vi "Vision Processing.vi"(4 "error in (no error)":errorcluster, 6 "CameraDevRef":T1) -> ()   [LabVIEW 2011]
uses:
  <vilib>/Rock Robotics/WPI/Camera/WPI_CameraDevRef.ctl
  Robot Global Data.vi
  <vilib>/vision/NI_Vision_Development_Module.lvlib
panel:
  in  "Scale":dbl=0.85
  in  "Minimum Power":dbl=0.23
  out "Aspect Ratio":dbl[](array[numeric])
  out "Offset":dbl
  in  "Max Distance for 1 hoop":dbl=8.0
  out "Raw Turret":dbl
  in  "Run Calculations":bool=TRUE
  out "Target X Coord":dbl
  out "Target Distance":dbl
  out "Target Y Coord":dbl
  out "Distance Array":dbl[](array[numeric])
  in  "Dead Band":dbl=0.09
  out "Number of Rectangles Visible":dbl
  out "Y Position Array":dbl[](array[numeric])
  out "X Position Array":dbl[](array[numeric])
  in  "View":bool
  out "Target Info":T2(array[cluster])
  in  "Area Size Limit":i32=444
  in  "Particle Count Limit":i32=8
  in  "Score Limits":T3={"Rect Coverage"=76.0, "Aspect Ratio"=40.0, "X Edge Strength"=40.0, "Y Edge Strength"=60.0}
  in  "Processing":enum32{"Color", "Intensity", "Intensity Open"}(tab)=enum."Intensity"
  in  "Luminance":i32=255
  in  "Saturation":i32=255
  in  "Hue":i32(knob)=65 scale=0.0..255.0
  in  "Margins":cluster{"Hue":i32, "Sat":i32, "Lum":i32}={"Hue"=20, "Sat"=27, "Lum"=30} {"Sat" scale=0.0..40.0; "Lum" scale=0.0..40.0; "Hue" scale=0.0..40.0}
  in  "Range":cluster{"Lower value":sgl, "Upper value":sgl}={"Lower value"=107.17391, "Upper value"=255.0} {"Lower value" scale=0.0..255.0; "Upper value" scale=0.0..255.0}
  in  "Range":cluster{"Lower value":sgl, "Upper value":sgl}={"Lower value"=123.804344, "Upper value"=255.0} {"Lower value" scale=0.0..255.0; "Upper value" scale=0.0..255.0}
  in  "View":bool
  out "Processed Image":T4(plugin-control)
  out "Original Image":T4(plugin-control)
  # "Instructions:\nProcessing the reflective tape that is illuminated by a ring light can be based\non color or light intensity.\nParticles within the image are scored by rectangle coverage, aspect ratio, and\nfor being hollow with a bold edge. A particle is considered a target if all scores\nare above the score limits. Particles can be annotated -- surrounded by\na rectangle and scores drawn to the left .\nTo control the number of particles being scored, use the count limit and the size\nlimit."
  # "(in)"
  # "To debug, Enable using the View button.\nFor color processing, you can click in the image to select the color for processing."
  # "Enable by clicking the View button.\nGreen scores are above the limit, orange are below. Inner/outer rect\nindicates all passed."
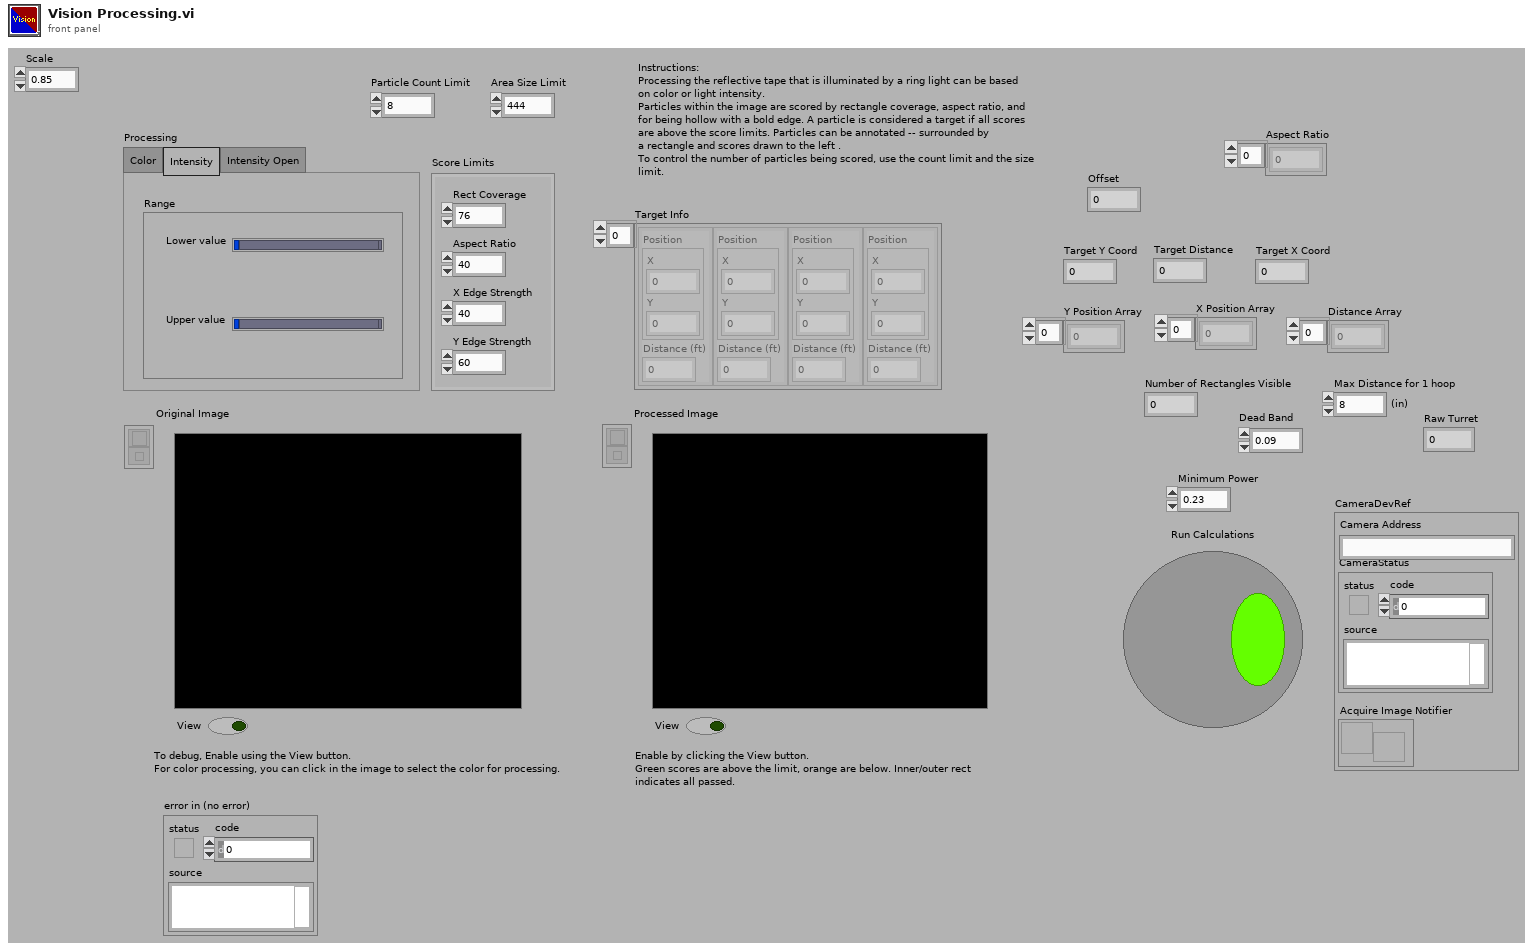
[diagram p1: front panel]
types:
  T1 = typedef "WPI_CameraDevRef.ctl" = cluster{"Camera Address":string, "CameraStatus":errorcluster, "Acquire Image Notifier":refnum<notifier>}
  T2 = cluster{"Position":cluster{"X":dbl, "Y":dbl}, "Distance (ft)":dbl}[]
  T3 = cluster{"Rect Coverage":dbl, "Aspect Ratio":dbl, "X Edge Strength":dbl, "Y Edge Strength":dbl}
  T4 = typedef "IMAQ Image.ctl" = refnum<image>
  T5 = typedef "Image Type" = u32
  T6 = enum32{"AutoM", "Close", "Dilate", "Erode", "Gradient", "Gradient out", "Gradient in", "Hit miss", "Open", "PClose", "POpen", "Thick", "Thin"}
  T7 = typedef "WPI_CameraImageSize.ctl" = enum16{"640x480", "320x240", "160x120"}
  T8 = cluster{"fps":i32, "compression":i32, "Image Size":T7}
  T9 = cluster{cluster{"Left":dbl, "Top":dbl, "Right":dbl, "Bottom":dbl}, dbl[]}[]
  T10 = cluster{"Left":dbl, "Top":dbl, "Right":dbl, "Bottom":dbl}
  T11 = cluster{"Target Center (-1 to 1)":cluster{"X":dbl, "Y":dbl}, "Distance (ft)":dbl}
  T12 = cluster{"Target Center (-1 to 1)":cluster{"X":dbl, "Y":dbl}, "Distance (ft)":dbl}[]
  T13 = typedef "WPI_JoystickDevRef.ctl" = cluster{"Device":T14}
  T14 = typedef "WPI_JoystickDeviceEnum.ctl" = enum16{"USB 1", "USB 2", "USB 3", "USB 4", "Kinect 1", "Kinect 2"}
  T15 = typedef "WPI_JoystickButtonState.ctl" = cluster{"Button 1":bool, "Button 2":bool, "Button 3":bool, "Button 4":bool, "Button 5":bool, "Button 6":bool, "Button 7":bool, "Button 8":bool, "Button 9":bool, "Button 10":bool, "Button 11":bool, "Button 12":bool}
  T16 = cluster{"axis 1 (x)":dbl, "axis 2 (y)":dbl, "axis 3 (throttle)":dbl, "axis 4":dbl, "axis 5":dbl, "axis 6":dbl}
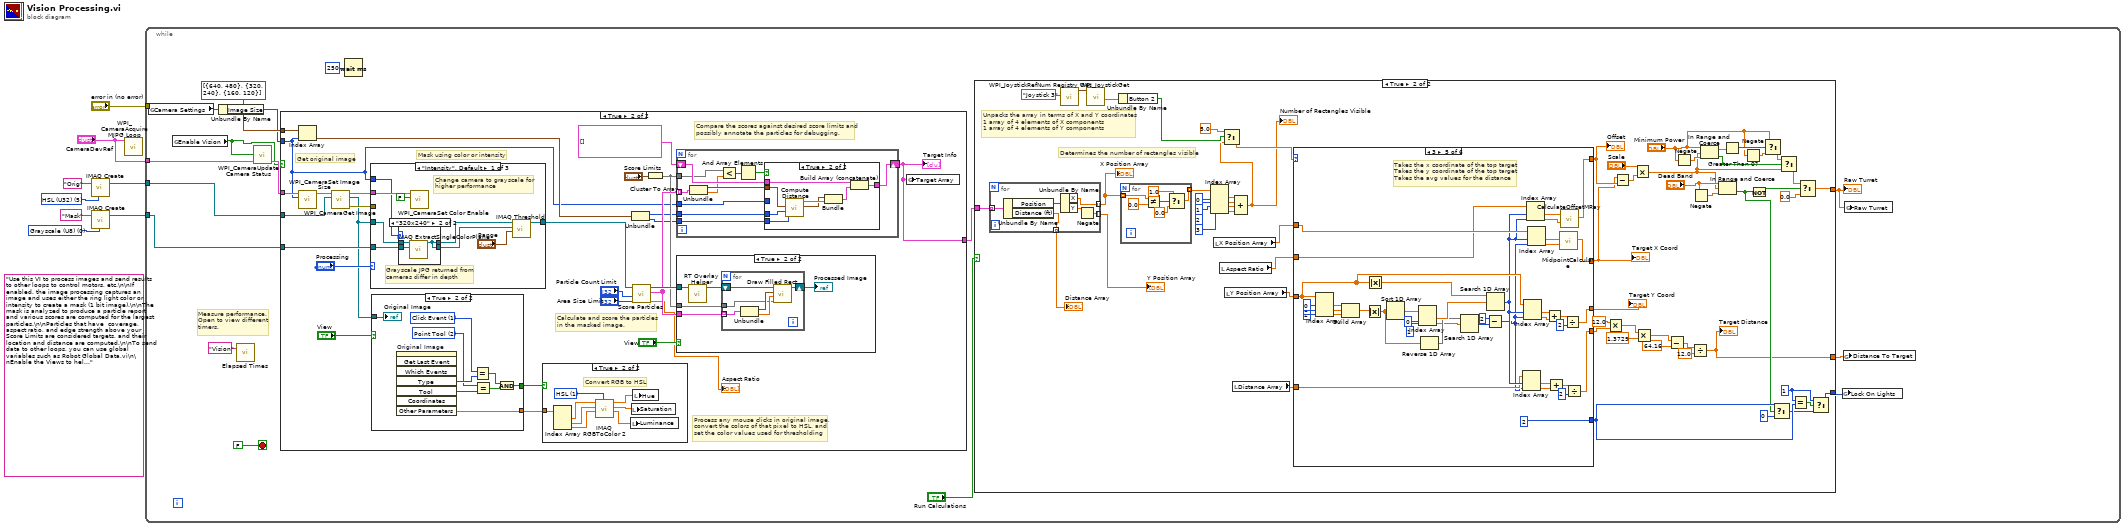
[diagram p0: block diagram]
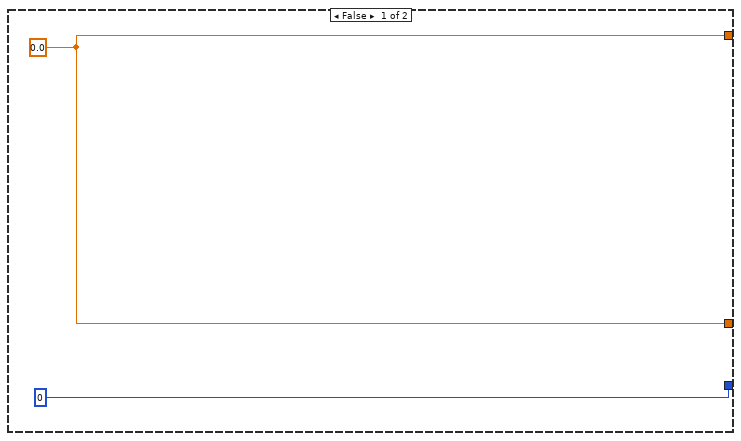
[diagram p2: hidden frame]
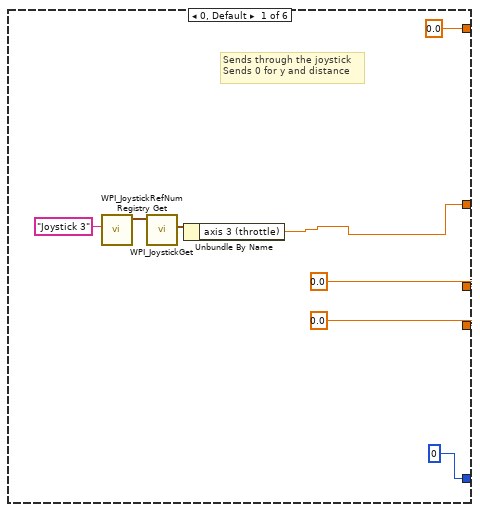
[diagram p3: hidden frame]
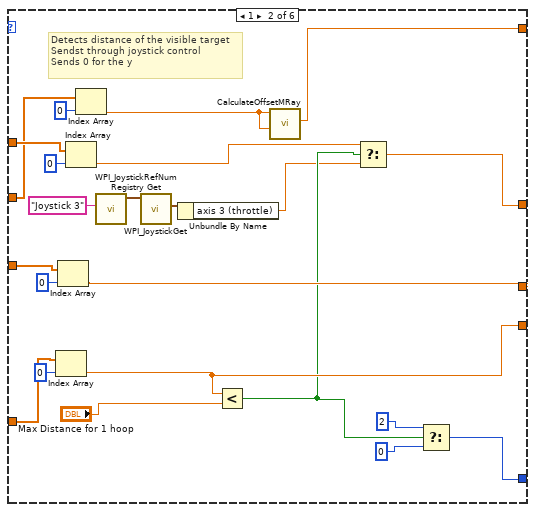
[diagram p4: hidden frame]
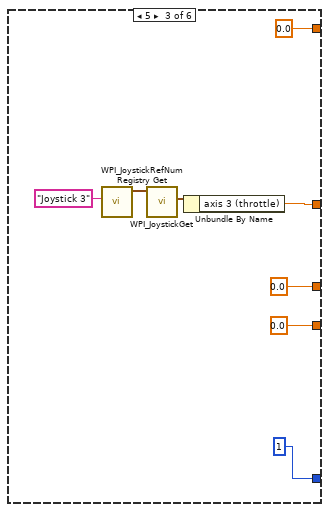
[diagram p5: hidden frame]
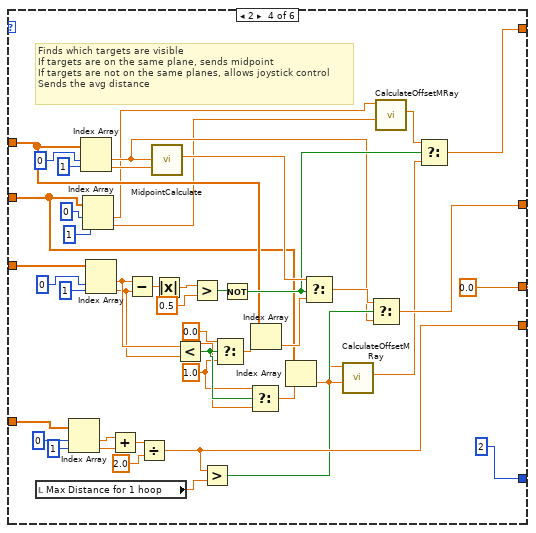
[diagram p6: hidden frame]
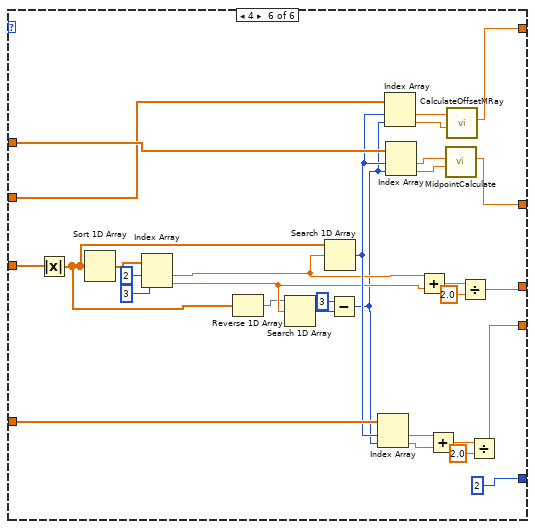
[diagram p7: hidden frame]
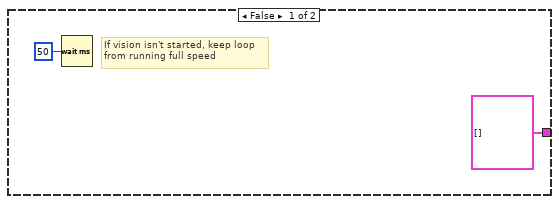
[diagram p8: hidden frame]
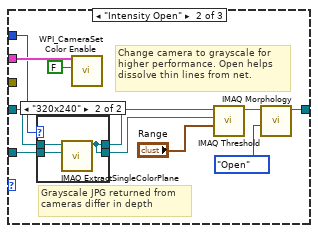
[diagram p11: hidden frame]
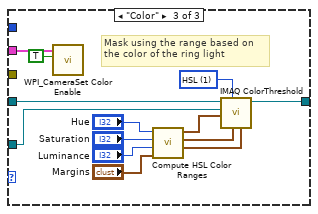
[diagram p13: hidden frame]
diagram:
  w3 = T5 0 items=["Grayscale (U8)", "Grayscale (I16)", "Grayscale (SGL)", "Complex (CSG)", "RGB (U32)", "HSL (U32)", "RGB (U64)", "Grayscale (U16)"] ("Image Type")
  (unwired) "Use this VI to process images and send results to other loops to control motors, etc.\n\nIf enabled, the image processing captures an image and uses either the ring light color or intensity to create a mask (1 bit image).\n\nThe mask is analyzed to produce a particle report and various scores are computed for the largest particles.\n\nParticles that have  coverage, aspect ratio, and edge strength above your Score Limits are considered targets, and their location and distance are computed.\n\nTo send data to other loops, you can use global variables such as Robot Global Data.vi\n\nEnable the Views to help debug color settings. Disable the View to speed up processing."
  w7 = T5 5 items=["Grayscale (U8)", "Grayscale (I16)", "Grayscale (SGL)", "Complex (CSG)", "RGB (U32)", "HSL (U32)", "RGB (U64)", "Grayscale (U16)"] ("Image Type")
  n1 = call "IMAQ Create"("Image Name"="Orig", "Image Type"=w7) -> ("New Image"=w6:T4)  [unwired: 2 in, 2 out]
  n2 = call "IMAQ Create"("Image Name"="Mask", "Image Type"=w3) -> ("New Image"=w1:T4)  [unwired: 2 in, 2 out]
  n3 = call <vilib>:"WPI_CameraAcquire MJPG Loop.vi"("CameraDevRef"="CameraDevRef") -> ()  [unwired: 11 in]
  n4 = while {
    tunnel: w6 -> [w23]
    tunnel: "CameraDevRef" -> [w22]
    tunnel: "error in (no error)" -> [_]
    tunnel: w1 -> [w18]
    stop <- FALSE stop-if-true
    # "Measure performance.\nOpen to view different\ntimers."
    n5 = global read "Robot Global Data.vi" "Camera Settings"() -> (w16:T8)
    n6 = global read "Robot Global Data.vi" "Enable Vision"() -> (w20:bool)
    n7 = Unbundle By Name(w16) -> ("Image Size"=w15:T7)
    n8 = call "Elapsed Times.vi"("Call Name"="Vision") -> ()  [unwired: 2 in, 1 out]
    n9 = call <vilib>:"WPI_CameraUpdate Camera Status.vi"("CameraDevRef In"=w22, "Enable Vision"=w20) -> ("CameraDevRef Out"=w21:T1)  [unwired: 3 in]
    n10 = case shown="True" w20 {
      tunnel: w23 -> [_ w271]
      tunnel: w21 -> [_ w267]
      tunnel: w18 -> [_ w258]
      tunnel: cluster{i32, i32}[] [{640, 480}, {320, 240}, {160, 120}] -> [_ w262]
      tunnel: w15 -> [_ w255]
      tunnel: [T2 [] w256] -> w14
      frame False {
        # "If vision isn't started, keep loop\nfrom running full speed"
        n11 = Wait (ms)(milliseconds to wait=u32 50) -> ()  [unwired: 1 out]
      }
      frame True {
        # "Compare the scores against desired score limits and\npossibly annotate the particles for debugging."
        # "Process any mouse clicks in original image,\nconvert the colors of that pixel to HSL, and\nset the color values used for thresholding"
        # "Calculate and score the particles\nin the masked image."
        # "Mask using color or intensity"
        # "Get original image"
        n12 = call <vilib>:"WPI_CameraSet Image Size.vi"("Image Size"=w255, "CameraDevRef"=w267) -> ("CameraDevRef Out"=w268:T1)  [unwired: 8 in, 1 out]
        n13 = Index Array(array=w262, index=w255) -> (element=w259:cluster{i32, i32})
        n14 = call <vilib>:"WPI_CameraGet Image.vi"("Image"=w271, "CameraDevRef"=w268) -> ("error out"=w269:errorcluster, "Image Out"=w257:T4, "CameraDevRef Out"=w270:T1)  [unwired: 7 in]
        n15 = case shown="\"Intensity\", Default" "Processing" {
          tunnel: w257 -> [w293 w305 w331]
          tunnel: [w296 w310 w330] -> w265
          tunnel: w270 -> [w294 w308 w321]
          tunnel: w269 -> [_ _ _]
          tunnel: w258 -> [w292 w306 w319]
          tunnel: w255 -> [w291 w307 _]
          frame "Intensity", Default {
            # "Grayscale JPG returned from\ncameras differ in depth"
            # "Change camera to grayscale for\nhigher performance"
            n16 = case shown="\"320x240\"" w291 {
              tunnel: w293 -> [w299 w302]
              tunnel: w292 -> [w298 w301]
              tunnel: [w299 w300] -> w290
              tunnel: [w298 w300] -> w289
              frame "640x480", Default {
              }
              frame "320x240" {
                n17 = call "IMAQ ExtractSingleColorPlane"("Image Dst"=w301, "Image Src"=w302) -> ("Image Dst Out"=w300:T4)  [unwired: 8 in, 1 out]
              }
            }
            n18 = call <vilib>:"WPI_CameraSet Color Enable.vi"("Color Enabled"=FALSE, "CameraDevRef"=w294) -> ()  [unwired: 8 in, 2 out]
            n19 = call "IMAQ Threshold"("Range"="Range", "Image Dst"=w289, "Image Src"=w290) -> ("Image Dst Out"=w296:T4)  [unwired: 3 in, 5 out]
          }
          frame "Intensity Open" {
            # "Grayscale JPG returned from\ncameras differ in depth"
            # "Change camera to grayscale for\nhigher performance. Open helps\ndissolve thin lines from net."
            n20 = case shown="\"320x240\"" w307 {
              tunnel: w305 -> [w315 w318]
              tunnel: w306 -> [w314 w317]
              tunnel: [w315 w316] -> w304
              tunnel: [w314 w316] -> w303
              frame "640x480", Default {
              }
              frame "320x240" {
                n21 = call "IMAQ ExtractSingleColorPlane"("Image Dst"=w317, "Image Src"=w318) -> ("Image Dst Out"=w316:T4)  [unwired: 8 in, 1 out]
              }
            }
            n22 = call <vilib>:"WPI_CameraSet Color Enable.vi"("Color Enabled"=FALSE, "CameraDevRef"=w308) -> ()  [unwired: 8 in, 2 out]
            n23 = call "IMAQ Threshold"("Range"="Range", "Image Dst"=w303, "Image Src"=w304) -> ("Image Dst Out"=w311:T4)  [unwired: 3 in, 5 out]
            n24 = call "IMAQ Morphology"("Operation"=T6."Open", "Image Src"=w311) -> ("Image Dst Out"=w310:T4)  [unwired: 8 in, 1 out]
          }
          frame "Color" {
            w329 = u16 1 items=["RGB", "HSL", "HSV", "HSI"] ("Color Mode")
            # "Mask using the range based on\nthe color of the ring light"
            n25 = call <vilib>:"WPI_CameraSet Color Enable.vi"("Color Enabled"=TRUE, "CameraDevRef"=w321) -> ()  [unwired: 8 in, 2 out]
            n26 = call "Compute HSL Color Ranges.vi"("Margins"="Margins", "Luminance"="Luminance", "Saturation"="Saturation", "Hue"="Hue") -> ("Lum Range"=w326:cluster{i32, i32}, "Sat Range"=w327:cluster{i32, i32}, "Hue Range"=w328:cluster{i32, i32})  [unwired: 5 in]
            n27 = call "IMAQ ColorThreshold"("Blue or Luma or Val or Inten Range"=w326, "Green or Sat Range"=w327, "Color Mode"=w329, "Red or Hue Range"=w328, "Image Dst"=w319, "Image Src"=w331) -> ("Image Dst Out"=w330:T4)  [unwired: 4 in, 1 out]
          }
        }
        n28 = case shown="True" "View" {
          tunnel: w257 -> [_ w351]
          tunnel: [_ w346] -> w264
          tunnel: [_ w343] -> w263
          frame False {
          }
          frame True {
            w344 = 2 items=["None", "Selection Tool", "Point Tool", "Line Tool", "Rectangle Tool", "Oval Tool", "Polygon Tool", "ClosedFreehandTool", "Annulus Tool", "Rotated Rectangle Tool", "Zoom Tool", "Pan Tool", "Polyline Tool", "Freehand Tool"] ("Tool")
            w345 = 1 items=["No Event"=0, "Click Event"=1, "Draw Event"=2, "Size Event"=4, "Scroll Event"=5, "Double Click Event"=8] ("Type")
            n29 = invoke on="Original Image" class="ImageControl" method="Get Last Event"() -> ("Type"=w347:i32, "Tool"=w350:i32, "Other Parameters"=w343:sgl[])  [unwired: 8 in, 5 out]
            n30 = Equal?(x=w345, y=w347) -> (x = y?=w348:bool)
            n31 = Equal?(x=w344, y=w350) -> (x = y?=w349:bool)
            n32 = And(x=w348, y=w349) -> (x .and. y?=w346:bool)
            "Original Image" <- w351
          }
        }
        n33 = case shown="True" w264 {
          tunnel: w263 -> [_ w288]
          frame False {
          }
          frame True {
            w287 = u16 1 items=["RGB", "HSL", "HSV", "HSI", "CIE L*a*b*", "CIE XYZ"] ("Color Mode")
            # "Convert RGB to HSL"
            n34 = Index Array(array=w288) -> (element #1=w286:sgl, element #2=w284:sgl, element #3=w282:sgl)  [unwired: 3 in]
            n35 = call "IMAQ RGBToColor 2"("Color Mode"=w287, "Blue value"=w282, "Green value"=w284, "Red value"=w286) -> ("Blue or Luma or Val or Inten or Z or b*value"=w281:dbl, "Green or Sat or Y or a* value"=w283:dbl, "Red or Hue or X or L* value"=w285:dbl)  [unwired: 4 in, 1 out]
            n36 = local write "Luminance"(w281) -> ()
            n37 = local write "Saturation"(w283) -> ()
            n38 = local write "Hue"(w285) -> ()
          }
        }
        n39 = Unbundle(w259) -> (w261:i32, w260:i32)
        n40 = call "Score Particles.vi"("Area Size Limit"="Area Size Limit", "Particle Count Limit"="Particle Count Limit", "Image Refnum in"=w265) -> ("Aspect Ratio"=→"Aspect Ratio":dbl[], "Scored Particle Info"=w276:T9, "Image Refnum out"=w279:T4)  [unwired: 6 in]
        n41 = Cluster To Array(cluster="Score Limits") -> (array=w274:dbl[])
        n42 = for {
          shift-right: [w361] -> w256
          shift-left: T2 [] -> [w362]
          tunnel: w261 -> [w360]
          tunnel: w276 -> [w358] mode=indexing
          tunnel: w274 -> [w353]
          tunnel: w255 -> [w357]
          tunnel: w260 -> [w352]
          n43 = Unbundle(w358) -> (w359:T10, w354:dbl[])
          n44 = Less?(x=w353, y=w354) -> (x < y?=w356:bool[])
          n45 = And Array Elements(Boolean array=w356) -> (logical AND=w355:bool)
          n46 = case shown="True" w355 {
            tunnel: w362 -> [w363 w371]
            tunnel: [w363 w370] -> w361
            tunnel: w359 -> [_ w366]
            tunnel: w360 -> [_ w368]
            tunnel: w357 -> [_ _]
            tunnel: w352 -> [_ w365]
            frame False {
            }
            frame True {
              n47 = call "Compute Distance.vi"("Y Image Resolution"=w365, "X Image Resolution"=w368, "Bounding Box"=w366) -> ("Target Center (-1 to 1)"=w364:cluster{"X":dbl, "Y":dbl}, "Distance (ft)"=w367:dbl)  [unwired: 7 in]
              n48 = Bundle("Target Center (-1 to 1)"=w364, "Distance (ft)"=w367) -> (w369:T11)  [unwired: 1 in]
              n49 = Build Array (concatenate)(w371, w369) -> (w370:T12)
            }
          }
        }
        "Target Info" <- w256
        n50 = case shown="True" "View" {
          tunnel: w279 -> [_ w333]
          tunnel: w276 -> [_ w335]
          tunnel: w274 -> [_ w334]
          frame False {
          }
          frame True {
            n51 = call "RT Overlay Helper.vi"("Refnum in"=w333) -> ("Refnum out"=w336:T4)  [unwired: 10 in]
            n52 = for {
              shift-right: [w341] -> w332
              shift-left: w336 -> [w342]
              tunnel: w335 -> [w338] mode=indexing
              tunnel: w334 -> [w337]
              n53 = Unbundle(w338) -> (w339:T10, w340:dbl[])
              n54 = call "Draw Filled Rect.vi"("Limits"=w337, "Scores"=w340, "Bounding Box"=w339, "image in"=w342) -> ("image out"=w341:T4)  [unwired: 7 in]
            }
            "Processed Image" <- w332
          }
        }
        n55 = global write "Robot Global Data.vi" "Target Array"(w256) -> ()
      }
    }
    n56 = Wait (ms)(milliseconds to wait=u32 250) -> ()  [unwired: 1 out]
    n57 = case shown="True" "Run Calculations" {
      tunnel: w14 -> [_ w66]
      tunnel: [w25 w36] -> w11
      tunnel: [0 ("f") w59] -> w10
      tunnel: [w25 w28] -> w9
      frame False {
        w25 = 0.0 ("f")
      }
      frame True {
        w60 = 1 ("y")
        # "Determines the number of rectangles visible"
        # "Unpacks the array in terms of X and Y coordinates\n1 array of 4 elements of X components\n1 array of 4 elements of Y components"
        n58 = for {
          tunnel: [w249] -> w67 mode=indexing
          tunnel: [w250] -> w77 mode=indexing
          tunnel: w66 -> [w247] mode=indexing
          tunnel: [w246] -> w80 mode=indexing
          n59 = Unbundle By Name(w247) -> ("Position"=w251:cluster{"X":dbl, "Y":dbl}, "Distance (ft)"=w246:dbl)
          n60 = Unbundle By Name(w251) -> ("X"=w250:dbl, "Y"=w248:dbl)
          n61 = Negate(x=w248) -> (-x=w249:dbl)
        }
        "X Position Array" <- w77
        "Y Position Array" <- w67
        "Distance Array" <- w80
        n62 = call <vilib>:"WPI_JoystickRefNum Registry Get.vi"("refnum name"="Joystick 3") -> ("JoystickDevRef"=w65:T13)  [unwired: 9 in, 1 out]
        n63 = call <vilib>:"WPI_JoystickGet.vi"("JoystickDevRef"=w65) -> ("Buttons"=w63:T15)  [unwired: 4 in, 2 out]
        n64 = Unbundle By Name(w63) -> ("Button 2"=w62:bool)
        n65 = for {
          tunnel: w77 -> [w90] mode=indexing
          tunnel: [w86] -> w76 mode=indexing
          n66 = Not Equal?(x=w90, y=0.0) -> (x != y?=w89:bool)
          n67 = Select(t=1.0, s=w89, f=0.0) -> (s? t:f=w86:dbl)
        }
        n68 = Index Array(array=w76, index #1=0 ("index"), index #2=1 ("index"), index #3=2 ("index"), index #4=3 ("index")) -> (element #1=w74:dbl, element #2=w75:dbl, element #3=w73:dbl, element #4=w72:dbl)
        n69 = local read "X Position Array"() -> (w78:dbl[])
        n70 = local read "Aspect Ratio"() -> (w54:dbl[])
        n71 = local read "Y Position Array"() -> (w82:dbl[])
        n72 = local read "Distance Array"() -> (w83:dbl[])
        n73 = Compound Arithmetic op=ADD(w74, w75, w73, w72) -> (w55:dbl)
        "Number of Rectangles Visible" <- w55
        n74 = Select(t=5.0, s=w62, f=w55) -> (s? t:f=w84:dbl)
        n75 = case shown="3" w84 {
          tunnel: w78 -> [_ w119 _ w139 w201 w241]
          tunnel: [w93 w113 w124 w149 w182 w237] -> w52
          tunnel: [0.0 ("X") w110 0.0 ("X") 0.0 ("X") w202 w236] -> w81
          tunnel: [0.0 ("X") w115 0.0 ("X") w152 w192 w231] -> w32
          tunnel: w82 -> [_ w111 _ w173 w197 w245]
          tunnel: w83 -> [_ w122 _ w161 w184 w240]
          tunnel: [0 w106 1 2 2 2] -> w58
          tunnel: [0.0 ("Offset") w103 0.0 ("Offset") w136 w189 w227] -> w53
          tunnel: w54 -> [_ w102 _ w131 w185 w223]
          frame 0, Default {
            # "Sends through the joystick\nSends 0 for y and distance"
            n76 = call <vilib>:"WPI_JoystickRefNum Registry Get.vi"("refnum name"="Joystick 3") -> ("JoystickDevRef"=w97:T13)  [unwired: 9 in, 1 out]
            n77 = call <vilib>:"WPI_JoystickGet.vi"("JoystickDevRef"=w97) -> ("Axes"=w95:T16)  [unwired: 4 in, 2 out]
            n78 = Unbundle By Name(w95) -> ("axis 3 (throttle)"=w93:dbl)
          }
          frame 1 {
            # "Detects distance of the visible target\nSendst through joystick control\nSends 0 for the y"
            n79 = Index Array(array=w122, index=0) -> (element=w115:dbl)
            n80 = Index Array(array=w111, index=0) -> (element=w110:dbl)
            n81 = Index Array(array=w119, index=0) -> (element=w104:dbl)
            n82 = Index Array(array=w102, index=0) -> (element=w100:dbl)
            n83 = call <vilib>:"WPI_JoystickRefNum Registry Get.vi"("refnum name"="Joystick 3") -> ("JoystickDevRef"=w118:T13)  [unwired: 9 in, 1 out]
            n84 = call <vilib>:"WPI_JoystickGet.vi"("JoystickDevRef"=w118) -> ("Axes"=w116:T16)  [unwired: 4 in, 2 out]
            n85 = Unbundle By Name(w116) -> ("axis 3 (throttle)"=w105:dbl)
            n86 = Less?(x=w115, y="Max Distance for 1 hoop") -> (x < y?=w108:bool)
            n87 = call "CalculateOffsetMRay.vi"("AR2"=w100, "AR1"=w100) -> ("Offset"=w103:dbl)  [unwired: 9 in]
            n88 = Select(t=w104, s=w108, f=w105) -> (s? t:f=w113:dbl)
            n89 = Select(t=2, s=w108, f=0) -> (s? t:f=w106:i32)
          }
          frame 5 {
            n90 = call <vilib>:"WPI_JoystickRefNum Registry Get.vi"("refnum name"="Joystick 3") -> ("JoystickDevRef"=w128:T13)  [unwired: 9 in, 1 out]
            n91 = call <vilib>:"WPI_JoystickGet.vi"("JoystickDevRef"=w128) -> ("Axes"=w126:T16)  [unwired: 4 in, 2 out]
            n92 = Unbundle By Name(w126) -> ("axis 3 (throttle)"=w124:dbl)
          }
          frame 2 {
            w142 = 1.0 ("f")
            w141 = 0.0 ("t")
            # "Finds which targets are visible\nIf targets are on the same plane, sends midpoint\nIf targets are not on the same planes, allows joystick control\nSends the avg distance"
            n93 = local read "Max Distance for 1 hoop"() -> (w151:dbl)
            n94 = Index Array(array=w161, index #1=0 ("index"), index #2=1 ("index")) -> (element #1=w160:dbl, element #2=w159:dbl)
            n95 = Index Array(array=w139, index #1=0 ("index"), index #2=1 ("index")) -> (element #1=w146:dbl, element #2=w145:dbl)
            n96 = Index Array(array=w131, index #1=0 ("index"), index #2=1 ("index")) -> (element #1=w133:dbl, element #2=w132:dbl)
            n97 = Index Array(array=w173, index #1=0 ("index"), index #2=1 ("index")) -> (element #1=w157:dbl, element #2=w156:dbl)
            n98 = Add(x=w160, y=w159) -> (x+y=w164:dbl)
            n99 = Subtract(x=w157, y=w156) -> (x-y=w170:dbl)
            n100 = Divide(x=w164, y=2.0) -> (x/y=w152:dbl)
            n101 = call "MidpointCalculate.vi"("X2"=w145, "X1"=w146) -> ("Midpoint"=w166:dbl)  [unwired: 9 in]
            n102 = Absolute Value(x=w170) -> (abs(x)=w169:dbl)
            n103 = Less?(x=w157, y=w156) -> (x < y?=w143:bool)
            n104 = Greater?(x=w169, y=0.5) -> (0:w167:bool)
            n105 = Greater?(x=w152, y=w151) -> (0:w150:bool)
            n106 = Select(t=w141, s=w143, f=w142) -> (s? t:f=w155:dbl)
            n107 = Not(x=w167) -> (.not. x?=w147:bool)
            n108 = Select(t=w142, s=w143, f=w141) -> (s? t:f=w140:dbl)
            n109 = Index Array(array=w139, index=w155) -> (element=w154:dbl)
            n110 = Index Array(array=w131, index=w140) -> (element=w138:dbl)
            n111 = Select(t=w166, s=w147, f=w154) -> (s? t:f=w148:dbl)
            n112 = call "CalculateOffsetMRay.vi"("AR2"=w138, "AR1"=w138) -> ("Offset"=w137:dbl)  [unwired: 9 in]
            n113 = Select(t=w148, s=w150, f=w146) -> (s? t:f=w149:dbl)
            n114 = call "CalculateOffsetMRay.vi"("AR2"=w132, "AR1"=w133) -> ("Offset"=w144:dbl)  [unwired: 9 in]
            n115 = Select(t=w144, s=w147, f=w137) -> (s? t:f=w136:dbl)
          }
          frame 3 {
            # "Takes the x coordinate of the top target\nTakes the y coordinate of the top target\nTakes the avg values for the distance"
            n116 = Index Array(array=w197, index #1=0 ("index"), index #2=1 ("index"), index #3=2 ("index")) -> (element #1=w212:dbl, element #2=w211:dbl, element #3=w210:dbl)
            n117 = Build Array(w212, w211, w210) -> (w209:dbl[])
            n118 = Absolute Value(x=w209) -> (abs(x)=w180:dbl[])
            n119 = Absolute Value(x=w197) -> (abs(x)=w200:dbl[])
            n120 = Sort 1D Array(array=w180) -> (sorted array=w208:dbl[])
            n121 = Index Array(array=w208, index #1=0 ("index"), index #2=1 ("index")) -> (element #1=w205:dbl, element #2=w178:dbl)
            n122 = Reverse 1D Array(array=w180) -> (reversed array=w179:dbl[])
            n123 = Search 1D Array(1D array=w179, element=w178) -> (index of element=w181:i32)  [unwired: 1 in]
            n124 = Subtract(x=2, y=w181) -> (x-y=w176:i32)
            n125 = Search 1D Array(1D array=w200, element=w205) -> (index of element=w188:i32)  [unwired: 1 in]
            n126 = Index Array(array=w184, index #1=w188, index #2=w176) -> (element #1=w194:dbl, element #2=w193:dbl)
            n127 = Index Array(array=w197, index #1=w188, index #2=w176) -> (element #1=w199:dbl, element #2=w198:dbl)
            n128 = Index Array(array=w185, index #1=w188, index #2=w188) -> (element #1=w187:dbl, element #2=w186:dbl)
            n129 = Index Array(array=w201, index #1=w188, index #2=w176) -> (element #1=w183:dbl, element #2=w190:dbl)
            n130 = Add(x=w199, y=w198) -> (x+y=w204:dbl)
            n131 = Add(x=w194, y=w193) -> (x+y=w195:dbl)
            n132 = call "MidpointCalculate.vi"("X2"=w190, "X1"=w183) -> ("Midpoint"=w182:dbl)  [unwired: 9 in]
            n133 = call "CalculateOffsetMRay.vi"("AR2"=w186, "AR1"=w187) -> ("Offset"=w189:dbl)  [unwired: 9 in]
            n134 = Divide(x=w204, y=2) -> (x/y=w202:dbl)
            n135 = Divide(x=w195, y=2) -> (x/y=w192:dbl)
          }
          frame 4 {
            n136 = Absolute Value(x=w245) -> (abs(x)=w219:dbl[])
            n137 = Sort 1D Array(array=w219) -> (sorted array=w244:dbl[])
            n138 = Index Array(array=w244, index #1=2 ("index"), index #2=3 ("index")) -> (element #1=w222:dbl, element #2=w221:dbl)
            n139 = Reverse 1D Array(array=w219) -> (reversed array=w220:dbl[])
            n140 = Search 1D Array(1D array=w220, element=w221) -> (index of element=w218:i32)  [unwired: 1 in]
            n141 = Search 1D Array(1D array=w219, element=w222) -> (index of element=w226:i32)  [unwired: 1 in]
            n142 = Subtract(x=3, y=w218) -> (x-y=w217:i32)
            n143 = Index Array(array=w240, index #1=w226, index #2=w217) -> (element #1=w233:dbl, element #2=w232:dbl)
            n144 = Index Array(array=w223, index #1=w226, index #2=w217) -> (element #1=w224:dbl, element #2=w225:dbl)
            n145 = Index Array(array=w241, index #1=w226, index #2=w217) -> (element #1=w229:dbl, element #2=w228:dbl)
            n146 = Add(x=w222, y=w221) -> (x+y=w239:dbl)
            n147 = Add(x=w233, y=w232) -> (x+y=w234:dbl)
            n148 = call "MidpointCalculate.vi"("X2"=w228, "X1"=w229) -> ("Midpoint"=w237:dbl)  [unwired: 9 in]
            n149 = call "CalculateOffsetMRay.vi"("AR2"=w225, "AR1"=w224) -> ("Offset"=w227:dbl)  [unwired: 9 in]
            n150 = Divide(x=w239, y=2.0) -> (x/y=w236:dbl)
            n151 = Divide(x=w234, y=2.0) -> (x/y=w231:dbl)
          }
        }
        "Target Y Coord" <- w81
        "Target X Coord" <- w52
        "Offset" <- w53
        n152 = Multiply(x=12.0, y=w32) -> (x*y=w31:dbl)
        n153 = Subtract(x=w52, y=w53) -> (x-y=w47:dbl)
        n154 = Multiply(x="Scale", y=w47) -> (x*y=w38:dbl)
        n155 = Multiply(x=w31, y=1.3729) -> (x*y=w49:dbl)
        n156 = Subtract(x=w49, y=64.16) -> (x-y=w29:dbl)
        n157 = Negate(x="Minimum Power") -> (-x=w45:dbl)
        n158 = Divide(x=w29, y=12.0) -> (x/y=w28:dbl)
        "Target Distance" <- w28
        n159 = Negate(x="Dead Band") -> (-x=w79:dbl)
        n160 = In Range and Coerce(upper limit="Minimum Power", x=w38, lower limit=w45) -> (coerced(x)=w41:dbl, In Range?=w42:bool)
        n161 = In Range and Coerce(upper limit="Dead Band", x=w38, lower limit=w79) -> (In Range?=w34:bool)  [unwired: 1 out]
        n162 = Greater Than 0?(x=w41) -> (x > 0?=w40:bool)
        n163 = Negate(x="Minimum Power") -> (-x=w37:dbl)
        n164 = Not(x=w34) -> (.not. x?=w35:bool)
        n165 = Select(t="Minimum Power", s=w40, f=w37) -> (s? t:f=w39:dbl)
        n166 = Select(t=w58, s=w34, f=0) -> (s? t:f=w56:i32)
        n167 = Select(t=w39, s=w42, f=w38) -> (s? t:f=w43:dbl)
        n168 = Equal?(x=w60, y=w58) -> (x = y?=w61:bool)
        n169 = Select(t=w43, s=w35, f=0.0) -> (s? t:f=w36:dbl)
        n170 = Select(t=w60, s=w61, f=w56) -> (s? t:f=w59:i32)
      }
    }
    "Raw Turret" <- w11
    n171 = global write "Robot Global Data.vi" "Lock On Lights"(w10) -> ()
    n172 = global write "Robot Global Data.vi" "Distance To Target"(w9) -> ()
    n173 = global write "Robot Global Data.vi" "Raw Turret"(w11) -> ()
  }
